vi "Normalize Channel.vi"(0 "Upper Threshold (% of Max)":dbl=80.0, 5 "Lower Threshold (% of Min)":dbl=120.0, 7 "index (row)":i32, 9 "data":dbl[][](array[numeric])) -> (4 "Upper Voltage Threshold":dbl, 6 "Lower Voltage Threshold":dbl, 8 "Channel Data":dbl[](array[numeric]), 10 "Normalized Max (Channel Max - Channel Min)":dbl, 15 "Number of Samples":i32)   [LabVIEW 2009]
uses:
  <vilib>/Analysis/NI_AALBase.lvlib
panel:
  out "Waveform Graph 2":dbl[][](graph)
  out "Waveform Graph":dbl[](graph)
  out "Lower Array Mean":dbl format="%0.2f"
  out "Upper Array Mean":dbl format="%0.2f"
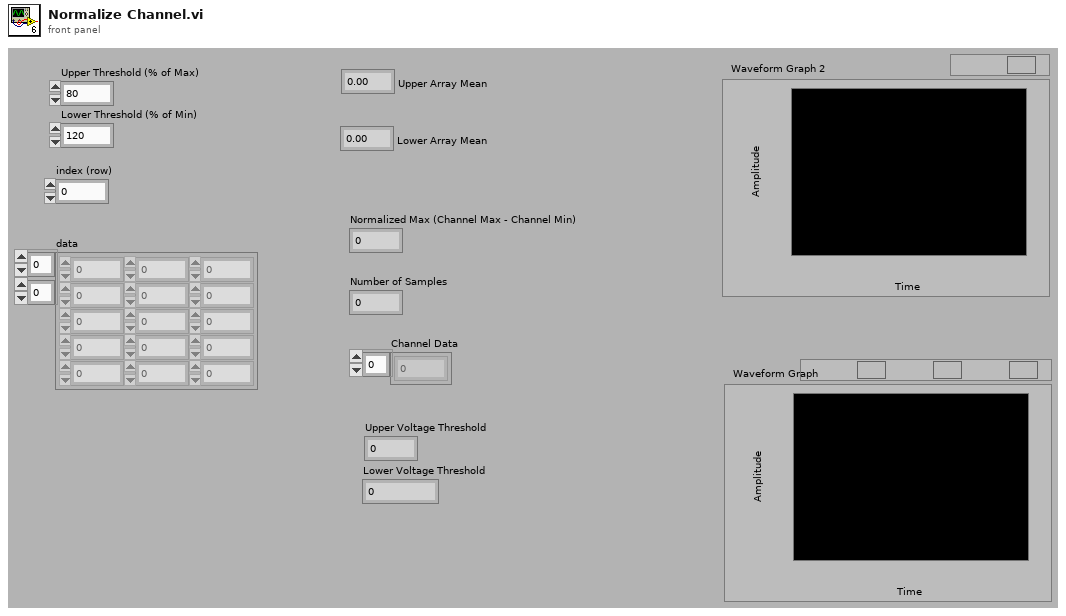
[diagram p1: front panel]
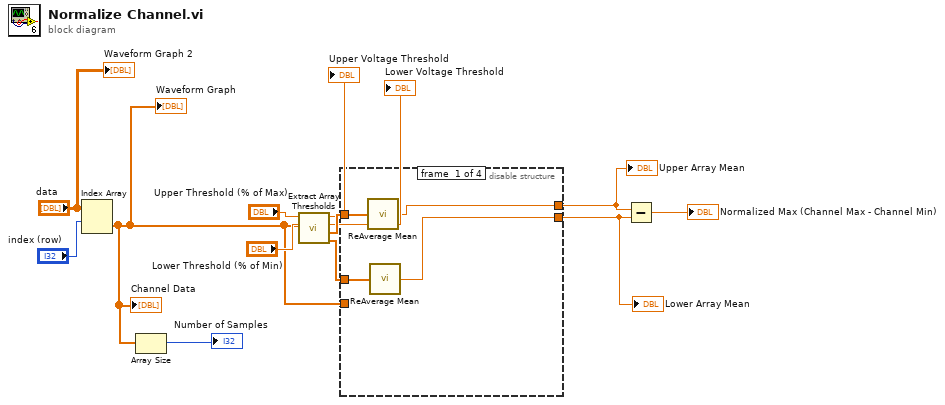
[diagram p0: block diagram]
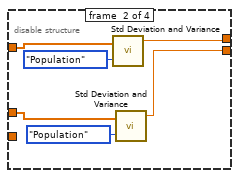
[diagram p2: hidden frame]
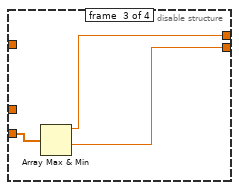
[diagram p3: hidden frame]
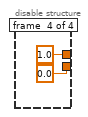
[diagram p4: hidden frame]
diagram:
  n1 = Index Array(array="data", index (row)="index (row)") -> (element=w2:dbl[])  [unwired: 1 in]
  "Channel Data" <- w2
  "Waveform Graph" <- w2
  n2 = Array Size(array=w2) -> (size(s)=→"Number of Samples":i32)
  n3 = call "Extract Array Thresholds.vi"("data"=w2, "Lower Threshold (% of Min)"="Lower Threshold (% of Min)", "Upper Threshold (% of Max)"="Upper Threshold (% of Max)") -> ("Lower  Subarray"=w5:dbl[], "Upper Subarray"=w6:dbl[], "Lower Voltage Threshold"=→"Lower Voltage Threshold":dbl, "Upper Voltage Threshold"=→"Upper Voltage Threshold":dbl)  [unwired: 5 in]
  n4 = disable-structure shown="Enabled" {
    disable-tunnel: w5 -> [w17 w18 _ _]
    disable-tunnel: w6 -> [w16 w19 _ _]
    disable-tunnel: [w15 w21 w25 1.0 ("Upper Array Mean")] -> w8
    disable-tunnel: [w14 w20 w24 0.0 ("Lower Array Mean")] -> w7
    disable-tunnel: w2 -> [_ _ w26 _]
    frame #0 {
      n5 = call "ReAverage Mean.vi"("Lower  Array"=w16) -> ("mean"=w15:dbl)
      n6 = call "ReAverage Mean.vi"("Lower  Array"=w17) -> ("mean"=w14:dbl)
    }
    frame #1 {
      n7 = call <vilib>:"Std Deviation and Variance.vi"("X"=w19, "Weighting (Sample)"=enum16{"Sample", "Population"}."Population") -> ("mean"=w21:dbl)  [unwired: 2 out]
      n8 = call <vilib>:"Std Deviation and Variance.vi"("X"=w18, "Weighting (Sample)"=enum16{"Sample", "Population"}."Population") -> ("mean"=w20:dbl)  [unwired: 2 out]
    }
    frame #2 {
      n9 = Array Max & Min(array=w26) -> (max value=w25:dbl, min value=w24:dbl)  [unwired: 2 out]
    }
    frame #3 {
    }
  }
  "Upper Array Mean" <- w8
  "Lower Array Mean" <- w7
  n10 = Subtract(x=w8, y=w7) -> (x-y=→"Normalized Max (Channel Max - Channel Min)":dbl)
  "Waveform Graph 2" <- "data"
